vi "Pre Launch Init.vi"(11 "IObserver in":refnum<class "IObserver.lvclass">) -> (0 "error out":errorcluster, 3 "IObserver out":refnum<class "IObserver.lvclass">)   [LabVIEW 2017, in "IObserver.lvlib" / "IObserver.lvclass"]
doc: "(<B>Filename</B>: Actor Framework.lvlib:Actor.lvclass:Pre Launch Init.vi)\n\nDefines behavior that occurs after the Launch Nested Actor method is invoked but before the actor's Actor Core method begins running.\n\nBy default, this method does nothing. A descendant class may override it to define behavior."
uses:
  IObserver.lvclass
  <vilib>/ActorFramework/Actor/Actor.lvclass
  gpm_packages/@cs/event-logger/Source/Composed Log/Types/Log Level.ctl
  gpm_packages/@cs/event-logger/Source/Composed Log/Composed Log.lvlib
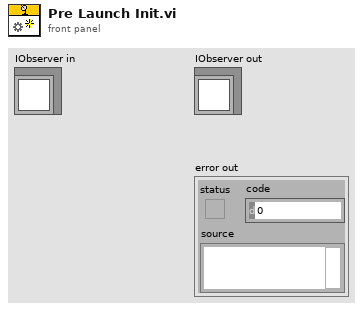
[diagram p1: front panel]
types:
  T1 = typedef "Composed Log.lvlib/Log Level.ctl" = enum16{"Debug", "Info", "Warning", "Error", "Critical"}
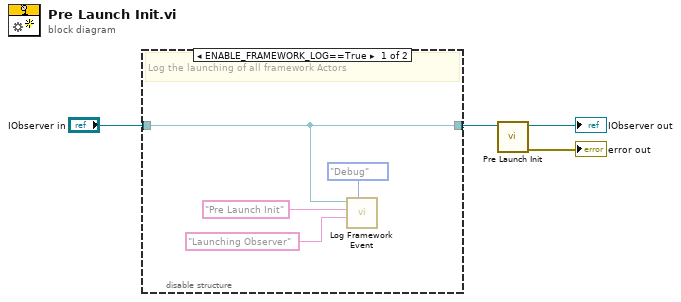
[diagram p0: block diagram]
diagram:
  n1 = disable-structure shown="ENABLE_FRAMEWORK_LOG==True" {
    disable-tunnel: "IObserver in" -> [w7 w9]
    disable-tunnel: [w7 w9] -> w1
    frame condition #0 {
      # "Log the launching of all framework Actors"
      n2 = call "Log Framework Event.vi"("Event Level (Debug)"=Log_Level."Debug", "Data To Log"="Launching Observer", "Caller Info (\"\")"="Pre Launch Init" ("Caller Info (\"\")"), "IObserver in"=w7) -> ()  [unwired: 7 in, 1 out]
    }
    frame condition #1 (active) {
      # "Remove all logging from this method at compile time"
    }
  }
  n3 = call-parent "Pre Launch Init.vi"("Actor in"=w1) -> ("error out"=→"error out":errorcluster, "Actor out"=→"IObserver out":refnum<class "IObserver.lvclass">)  [unwired: 9 in]
